vi "Engine Library Name.vi"() -> (3 "Engine Library Name":string)   [LabVIEW 2017, in "Data Sharing Framework Engine.lvlib"]
uses:
  Data Sharing Framework Engine.lvlib
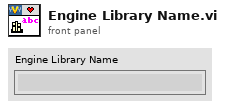
[diagram p1: front panel]
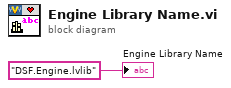
[diagram p0: block diagram]
diagram:
  "Engine Library Name" <- "DSF.Engine.lvlib" ("Library Name")
